vi "timing sensors.vi"(8 "error in":errorcluster) -> (0 "error out":errorcluster)   [LabVIEW 2020]
uses:
  <vilib>/robotics/Simulator/Engine/ctl/DeviceID.ctl
  Robot Global Data.vi
  <vilib>/Rock Robotics/Network Tables/NT Write Number.vi
  <instrlib>/Devantech SRF05/HAIOL/Devantech SRF05.lvclass
  <vilib>/robotics/Simulator/NI_Robotics_Simulator.lvlib
  <instrlib>/Devantech SRF05/HAIOL/Simulator/Devantech SRF05 Simulator.lvclass
panel:
  out "time (s)":dbl
  out "stop distance (cm)":dbl(graph)
  out "start distance (cm)":dbl(graph)
  # "This code is added just for the simulation timer.  It starts the timer when thr robot begins and stops the timer when the robot finishes the maze. \n\nIt is not expected that you would edit this code.  \n\nWhile this simulation project is not intended to run on a real robot, this code would be removed before building for the roboRIO target."
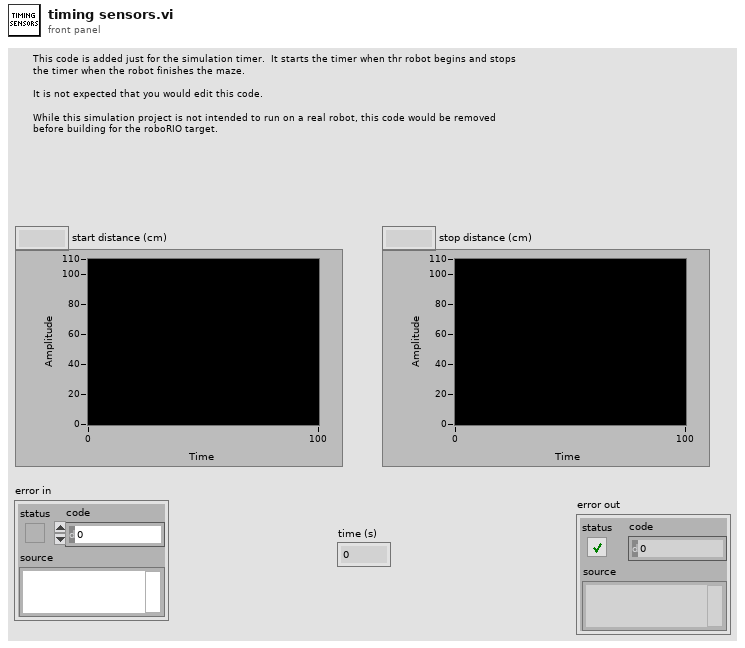
[diagram p1: front panel]
types:
  T1 = typedef "NI_Robotics_Simulator.lvlib/DeviceID.ctl" = cluster{"robot ID":string, "sensor/actuator ID":string}
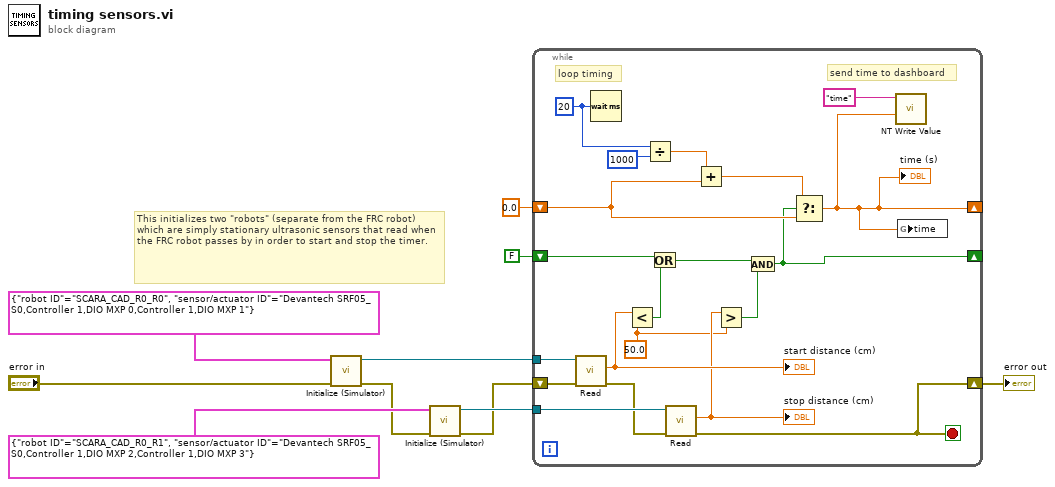
[diagram p0: block diagram]
diagram:
  # "This initializes two \"robots\" (separate from the FRC robot) which are simply stationary ultrasonic sensors that read when the FRC robot passes by in order to start and stop the timer."
  n1 = call <instrlib>:"Initialize (Simulator).vi"("error in (no error)"="error in", "Device ID"=T1 {"robot ID"="SCARA_CAD_R0_R0", "sensor/actuator ID"="Devantech SRF05_S0,Controller 1,DIO MXP 0,Controller 1,DIO MXP 1"}) -> ("error out"=w4:errorcluster, "Devantech SRF05 out"=w8:refnum<class "Devantech SRF05.lvclass">)  [unwired: 8 in]
  n2 = call <instrlib>:"Initialize (Simulator).vi"("error in (no error)"=w4, "Device ID"=T1 {"robot ID"="SCARA_CAD_R0_R1", "sensor/actuator ID"="Devantech SRF05_S0,Controller 1,DIO MXP 2,Controller 1,DIO MXP 3"}) -> ("error out"=w3:errorcluster, "Devantech SRF05 out"=w6:refnum<class "Devantech SRF05.lvclass">)  [unwired: 8 in]
  n3 = while {
    tunnel: w8 -> [w30]
    shift-right: [w26] -> w7
    shift-left: w3 -> [w29]
    tunnel: w6 -> [w28]
    shift-right: [w14] -> _
    shift-left: FALSE -> [w24]
    shift-right: [w11] -> _
    shift-left: 0.0 -> [w21]
    stop <- w26 stop-if-true
    w19 = u32 20 ("milliseconds to wait")
    w15 = 50.0 ("y")
    # "loop timing"
    # "send time to dashboard"
    n4 = call-dynamic "Read.vi"("error in (no error)"=w29, "Devantech SRF05 in"=w30) -> ("error out"=w27:errorcluster, "Distance (cm)"=w25:dbl)  [unwired: 6 in, 2 out]
    "start distance (cm)" <- w25
    n5 = Wait (ms)(milliseconds to wait=w19) -> ()  [unwired: 1 out]
    n6 = Less?(x=w25, y=w15) -> (x < y?=w23:bool)
    n7 = Divide(x=w19, y=u32 1000) -> (x/y=w17:dbl)
    n8 = Or(x=w24, y=w23) -> (x .or. y?=w22:bool)
    n9 = call-dynamic "Read.vi"("error in (no error)"=w27, "Devantech SRF05 in"=w28) -> ("error out"=w26:errorcluster, "Distance (cm)"=w16:dbl)  [unwired: 6 in, 2 out]
    "stop distance (cm)" <- w16
    n10 = Add(x=w17, y=w21) -> (x+y=w20:dbl)
    n11 = Greater?(x=w16, y=w15) -> (0:w13:bool)
    n12 = And(x=w22, y=w13) -> (x .and. y?=w14:bool)
    n13 = Select(t=w20, s=w14, f=w21) -> (s? t:f=w11:dbl)
    "time (s)" <- w11
    n14 = call-poly <vilib>:"NT Write Value.vi"("Numeric"=w11, "Name"="time") -> ()  [unwired: 9 in, 1 out]
    n15 = global write "Robot Global Data.vi" "time"(w11) -> ()
  }
  "error out" <- w7
